vi "GetTotalSequenceSteps.vi"(8 "error in (no error)":errorcluster, 11 "VariableManagerRef in":refnum<vi>) -> (0 "error out":errorcluster, 2 "TotalSequenceSteps":i32, 3 "VariableManagerRef out":refnum<vi>)   [LabVIEW 2013, in "VariableManagerAPI.lvlib"]
doc: "An error is thrown if a sequence function cannot be evaluated."
uses:
  VariableManagerAPI.lvlib
  VariableManager/VariableManager.lvclass
  VariableValue/VariableValue.lvclass
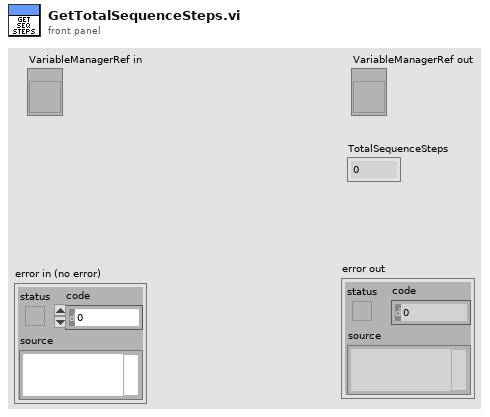
[diagram p1: front panel]
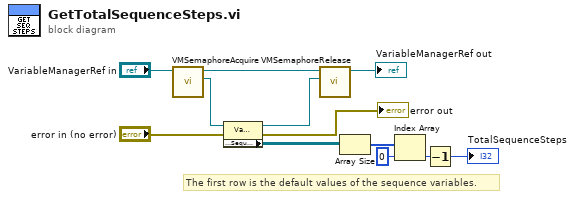
[diagram p0: block diagram]
diagram:
  # "The first row is the default values of the sequence variables."
  n1 = call "VMSemaphoreAcquire.vi"("VariableManagerRef in"="VariableManagerRef in") -> ("VariableManager"=w3:refnum<class "VariableManager.lvclass">, "VariableManagerRef out"=w11:refnum<vi>)  [unwired: 7 in, 2 out]
  n2 = property class="VariableManager.lvclass"(reference=w3, error in="error in (no error)") -> (reference out=w5:refnum<class "VariableManager.lvclass">, error out=→"error out":errorcluster, "Accessors:SequenceValues"=w9:refnum<class "VariableValue.lvclass">[][])
  n3 = call "VMSemaphoreRelease.vi"("VariableManager"=w5, "VariableManagerRef in"=w11) -> ("VariableManagerRef out"=→"VariableManagerRef out":refnum<vi>)  [unwired: 8 in, 1 out]
  n4 = Array Size(array=w9) -> (size(s)=w6:i32[])
  n5 = Index Array(array=w6, index=0) -> (element=w8:i32)
  n6 = Decrement(x=w8) -> (x-1=→"TotalSequenceSteps":i32)
